vi "takepressure2.vi"() -> ()   [LabVIEW 2011]
uses:
  <vilib>/Utility/file.llb/Write To Spreadsheet File (DBL).vi
panel:
  in  "Save Data File":path=path "C:/Documents and Settings/Helimak/My Documents/carterdodd/IonGauge/data.txt"
  out "Voltage Output":dynamicdata(graph)
  in  "Sample Rate":dbl=10.0
  in  "Sampling Time":dbl=60.0
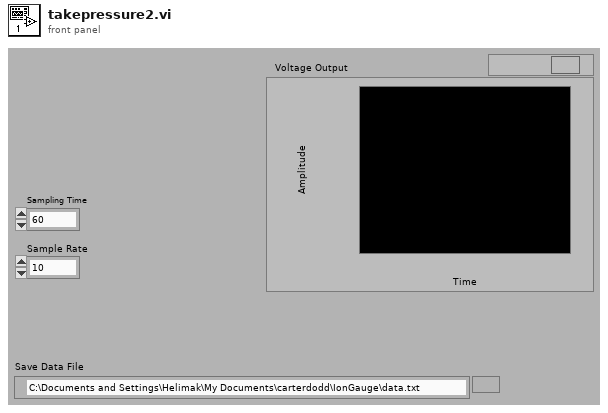
[diagram p1: front panel]
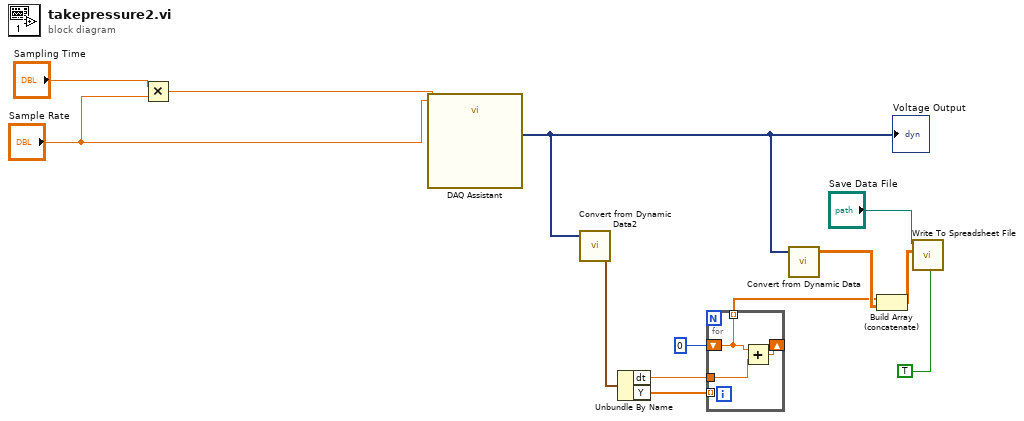
[diagram p0: block diagram]
diagram:
  n1 = Multiply(x="Sampling Time", y="Sample Rate") -> (x*y=w11:dbl)
  n2 = call "DAQ Assistant"("rate"="Sample Rate", "number of samples"=w11) -> ("data"=w7:dynamicdata)  [unwired: 15 in, 2 out]
  "Voltage Output" <- w7
  n3 = call "Convert from Dynamic Data2"("Dynamic Data Type"=w7) -> ("Waveform"=w6:waveform(dbl))  [unwired: 3 in]
  n4 = Unbundle By Name(w6) -> ("dt"=w5:dbl, "Y"=w4:dbl[])
  n5 = for {
    shift-right: [w15] -> _
    shift-left: 0 -> [w14]
    tunnel: w5 -> [w16]
    tunnel: [w14] -> w1 mode=indexing
    tunnel: w4 -> [_] mode=indexing
    n6 = Add(x=w14, y=w16) -> (x+y=w15:dbl)
  }
  n7 = call "Convert from Dynamic Data"("Dynamic Data Type"=w7) -> ("Array"=w2:dbl[][])  [unwired: 3 in]
  n8 = Build Array (concatenate)(w1, w2) -> (w3:dbl[][])
  n9 = call-poly <vilib>:"Write To Spreadsheet File.vi"("transpose? (no:F)"=TRUE, "2D data"=w3, "file path (dialog if empty)"="Save Data File") -> ()  [unwired: 5 in, 1 out]
